vi "Write configuration item.vi"(8 "error in (no error)":errorcluster, 9 "Value":string, 10 "Name in":string, 11 "IConfigDBQueries in":refnum<class "mysql-queries.lvclass">) -> (0 "error out":errorcluster, 2 "Query":string)   [LabVIEW 2020, in "mysql-queries.lvlib" / "mysql-queries.lvclass"]
uses:
  mysql-queries.lvclass
  mysql-queries.lvclass/mysql-queries.ctl
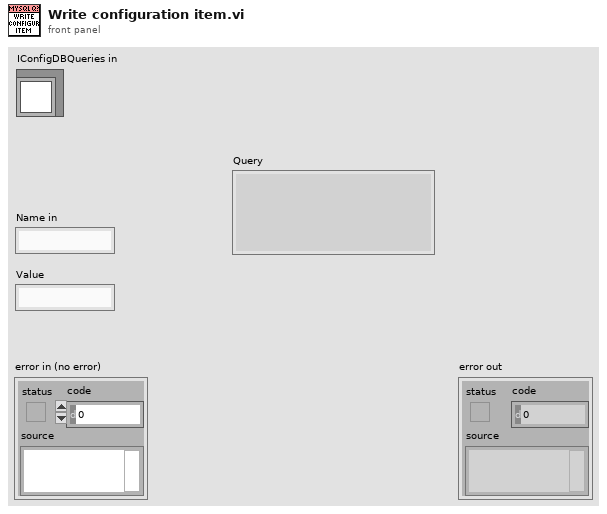
[diagram p1: front panel]
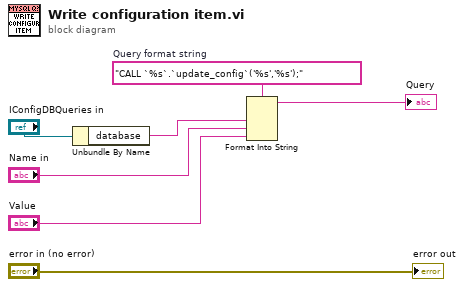
[diagram p0: block diagram]
diagram:
  w7 = "CALL `%s`.`update_config`('%s','%s');"  # Query format string
  n1 = Unbundle By Name("IConfigDBQueries in") -> ("database"=w5:string)
  n2 = Format Into String(format string=w7, w5, "Name in", "Value") -> (resulting string=→"Query":string)  [unwired: 2 in, 1 out]
  "error out" <- "error in (no error)"
